vi "gate sts with temp.vi"() -> ()   [LabVIEW 2010]
uses:
  <userlib>/Nanonis Prog Interface V5/Nanonis Prog Interface.lvlib
panel:
  out "Current Gate Voltage (V)":dbl
  out "Ender":bool
  out "Stop Loop":bool
  in  "Stop":bool
  in  "Increment Gate (V)":dbl
  in  "End Gate (V)":dbl
  in  "Start Gate (V)":dbl
  in  "Basename":string
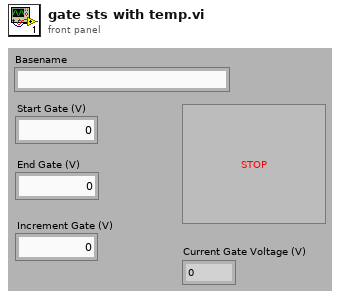
[diagram p1: front panel]
types:
  T1 = cluster{"Save all":enum16{"no change", "on", "off"}, "Number of Sweeps (0=no change)":i32}
  T2 = enum16{"Set Heater Voltage", "Read Heater Voltage", "Read Heater Current", "Read 1K Pot Temperature", "Read IVC Sorb Temperature", "Read Needle Valve Temperature", "Read Still Pressure", "Read Mixing Chamber Temperature", "Read STM RX Temperature", "Read STM CX Temperature", "Unstall Triton Loop", "Triton Stop", "Triton Stall Status"}
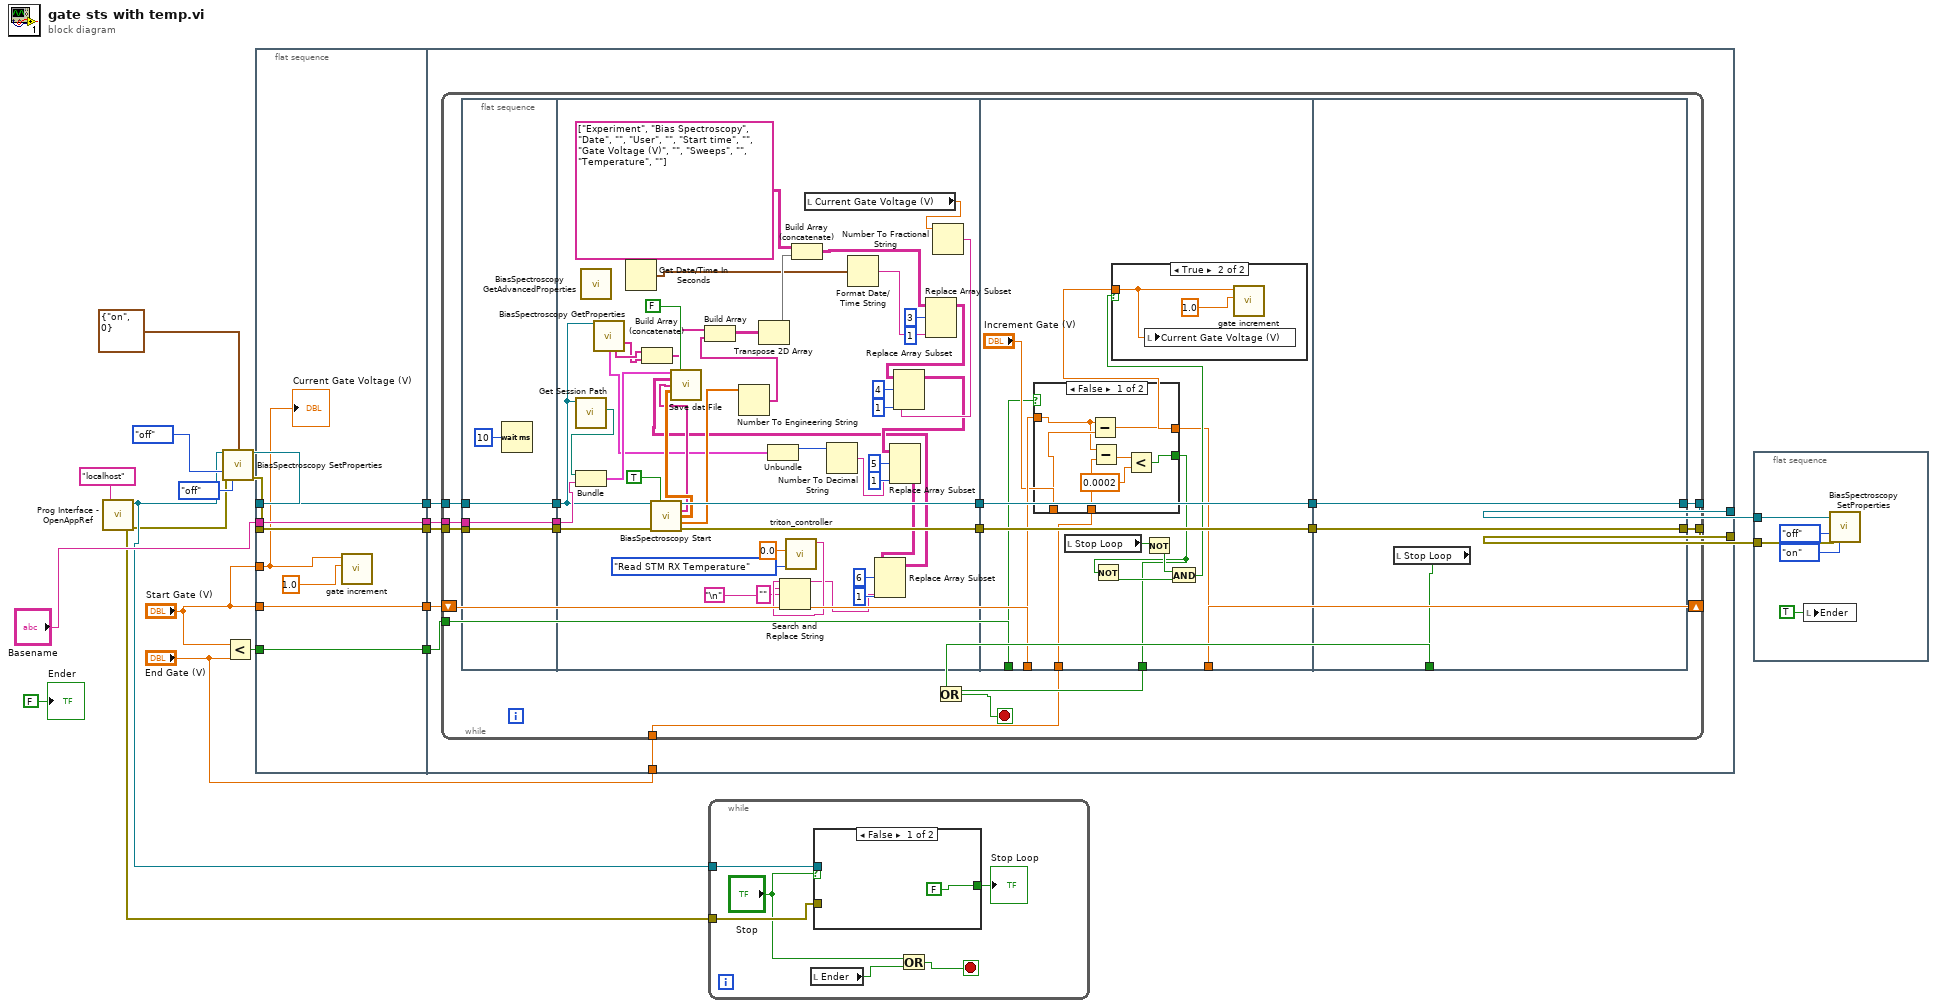
[diagram p0: block diagram]
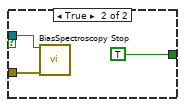
[diagram p2: hidden frame]
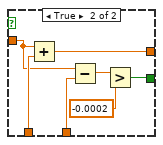
[diagram p3: hidden frame]
diagram:
  n1 = call <userlib>:"Prog Interface - OpenAppRef.vi"("Machine name (local machine IP)"="localhost" ("machine name (localhost)")) -> ("Error out"=w3:errorcluster, "Application reference"=w4:refnum<vi>)  [unwired: 5 in]
  n2 = call <userlib>:"BiasSpectroscopy SetProperties.vi"("Application ref in"=w4, "Autosave (no change)"=enum16{"no change", "on", "off"}."off", "Error in (no error)"=w3, "Save dialog"=enum16{"no change", "on", "off"}."off", "Multiple sweeps config"=T1 {"Save all"=enum."on", "Number of Sweeps (0=no change)"=0}) -> ("Application ref out"=w17:refnum<vi>, "Error out"=w18:errorcluster)  [unwired: 9 in]
  n3 = Less?(x="Start Gate (V)", y="End Gate (V)") -> (x < y?=w12:bool)
  n4 = flat-sequence {
    tunnel: "Start Gate (V)" -> [w23]
    tunnel: w12 -> [w24]
    tunnel: w17 -> [w25]
    tunnel: w18 -> [w26]
    tunnel: "Basename" -> [w27]
    tunnel: [w27] -> w11
    tunnel: [w26] -> w10
    tunnel: [w25] -> w9
    tunnel: [w24] -> w8
    tunnel: [w23] -> w7
    tunnel: "Start Gate (V)" -> [w21]
    tunnel: [w32] -> w15
    tunnel: [w31] -> w14
    tunnel: w11 -> [w35]
    tunnel: w10 -> [w34]
    tunnel: w9 -> [w33]
    tunnel: w8 -> [w30]
    tunnel: w7 -> [w29]
    tunnel: "End Gate (V)" -> [w28]
    frame #0 {
      n5 = call "gate increment.vi"("Increment"=1.0, "Gate Voltage"=w21) -> ()  [unwired: 10 in]
      "Current Gate Voltage (V)" <- w21
    }
    frame #1 {
      n6 = while {
        tunnel: w35 -> [w54]
        tunnel: w34 -> [w53]
        tunnel: w33 -> [w52]
        tunnel: [w51] -> w32
        tunnel: [w50] -> w31
        tunnel: w30 -> [w36]
        shift-right: [w40] -> _
        shift-left: w29 -> [w38]
        tunnel: w28 -> [w37]
        stop <- w41 stop-if-true
        n7 = flat-sequence {
          tunnel: w52 -> [w56]
          tunnel: w53 -> [w57]
          tunnel: w54 -> [w58]
          tunnel: [w58] -> w45
          tunnel: [w57] -> w44
          tunnel: [w56] -> w43
          tunnel: [w101] -> w47
          tunnel: [w102] -> w46
          tunnel: w45 -> [w94]
          tunnel: w44 -> [w103]
          tunnel: w43 -> [w93]
          tunnel: [w115] -> w49
          tunnel: [w114] -> w48
          tunnel: w47 -> [w115]
          tunnel: w46 -> [w114]
          tunnel: [w110] -> w40
          tunnel: [w108] -> w39
          tunnel: w38 -> [w107]
          tunnel: w37 -> [w105]
          tunnel: w36 -> [w104]
          tunnel: [w133] -> w51
          tunnel: [w134] -> w50
          tunnel: w49 -> [w134]
          tunnel: w48 -> [w133]
          tunnel: [w132] -> w42
          frame #0 {
            n8 = Wait (ms)(milliseconds to wait=u32 10) -> ()  [unwired: 1 out]
          }
          frame #1 {
            n9 = call <userlib>:"Get Session Path.vi"("Application ref in"=w93) -> ("Session path"=w99:path)  [unwired: 8 in, 2 out]
            n10 = Bundle("Session path"=w99, "Basename"=w94) -> (w98:cluster{"Session path":path, "Basename":string})  [unwired: 1 in]
            n11 = call <userlib>:"BiasSpectroscopy GetAdvancedProperties.vi"() -> ()  [unwired: 10 in, 6 out]
            n12 = call <userlib>:"BiasSpectroscopy GetProperties.vi"("Application ref in"=w93) -> ("Parameters"=w85:string[], "Multiple sweeps configuration"=w74:cluster{"Number of Sweeps":i32, "Save all":bool}, "Fixed parameters"=w86:string[])  [unwired: 7 in, 5 out]
            n13 = Get Date/Time In Seconds() -> (seconds since 1Jan1904=w84:timestamp)
            n14 = Build Array (concatenate)(w86, w85) -> (w90:string[])
            n15 = call <userlib>:"BiasSpectroscopy Start.vi"("Application ref in"=w93, "Get data (F)"=TRUE, "Error in (no error)"=w103) -> ("Application ref out"=w102:refnum<vi>, "Channels"=w96:string[], "Data"=w97:sgl[][], "Parameters"=w92:sgl[], "Error out"=w101:errorcluster)  [unwired: 8 in]
            n16 = Number To Engineering String(4:w92) -> (0:w91:string[])  [unwired: 3 in]
            n17 = Build Array(w90, w91) -> (w89:string[][])
            n18 = Transpose 2D Array(2D array=w89) -> (transposed array=w87:string[][])
            n19 = Unbundle(w74) -> ("Number of Sweeps"=w73:i32)  [unwired: 1 out]
            n20 = call "triton_controller.vi"("Numerical Argument"=0.0, "Command"=T2."Read STM RX Temperature") -> ("Response"=w62:string)  [unwired: 9 in]
            n21 = Search and Replace String(input string=w62, search string="\n", replace string="" ("replace string (\"\")")) -> (result string=w59:string)  [unwired: 5 in, 3 out]
            n22 = Build Array (concatenate)(string[][] [["Experiment", "Bias Spectroscopy"], ["Date", ""], ["User", ""], ["Start time", ""], ["Gate Voltage (V)", ""], ["Sweeps", ""], ["Temperature", ""]] ("Attributes"), w87) -> (w83:string[][])
            n23 = local read "Current Gate Voltage (V)"() -> (w76:dbl)
            n24 = Number To Decimal String(number=w73) -> (decimal integer string=w69:string)  [unwired: 1 in]
            n25 = Format Date/Time String(seconds (now)=w84) -> (date/time string=w82:string)  [unwired: 2 in]
            n26 = Replace Array Subset(array=w83, new element=w82, index (row)=3, index (col)=1 ("disabled index (col)")) -> (w79:string[][])
            n27 = Number To Fractional String(number=w76) -> (F-format string=w75:string)  [unwired: 3 in]
            n28 = Replace Array Subset(array=w79, new element=w75, index (row)=4, index (col)=1 ("disabled index (col)")) -> (w72:string[][])
            n29 = Replace Array Subset(array=w72, new element=w69, index (row)=5, index (col)=1 ("disabled index (col)")) -> (w64:string[][])
            n30 = Replace Array Subset(array=w64, new element=w59, index (row)=6, index (col)=1) -> (w63:string[][])
            n31 = call <userlib>:"Save dat File.vi"("Filename control"=w98, "Show save dialog (T)"=FALSE, "Attributes"=w63, "Channels names"=w96, "Data"=w97) -> ()  [unwired: 7 in, 4 out]
          }
          frame #2 {
            n32 = case shown="False" w104 {
              tunnel: w107 -> [w120 w126]
              tunnel: "Increment Gate (V)" -> [w121 w129]
              tunnel: [w122 w128] -> w110
              tunnel: w105 -> [w119 w127]
              tunnel: [w117 w125] -> w108
              frame False {
                n33 = Subtract(x=w120, y=w121) -> (x-y=w122:dbl)
                n34 = Subtract(x=w120, y=w119) -> (x-y=w118:dbl)
                n35 = Less?(x=w118, y=0.0002) -> (x < y?=w117:bool)
              }
              frame True {
                n36 = Add(x=w126, y=w129) -> (x+y=w128:dbl)
                n37 = Subtract(x=w126, y=w127) -> (x-y=w124:dbl)
                n38 = Greater?(x=w124, y=-0.0002) -> (0:w125:bool)
              }
            }
            n39 = local read "Stop Loop"() -> (w113:bool)
            n40 = Not(x=w108) -> (.not. x?=w109:bool)
            n41 = Not(x=w113) -> (.not. x?=w111:bool)
            n42 = And(x=w111, y=w109) -> (x .and. y?=w112:bool)
            n43 = case shown="True" w112 {
              tunnel: w110 -> [_ w131]
              frame False {
              }
              frame True {
                n44 = local write "Current Gate Voltage (V)"(w131) -> ()
                n45 = call "gate increment.vi"("Increment"=1.0, "Gate Voltage"=w131) -> ()  [unwired: 10 in]
              }
            }
          }
          frame #3 {
            n46 = local read "Stop Loop"() -> (w132:bool)
          }
        }
        n47 = Or(x=w39, y=w42) -> (x .or. y?=w41:bool)
      }
    }
  }
  n48 = while {
    tunnel: w4 -> [w140]
    tunnel: w3 -> [w139]
    stop <- w136 stop-if-true
    n49 = local read "Ender"() -> (w135:bool)
    n50 = case shown="False" "Stop" {
      tunnel: w140 -> [_ w144]
      tunnel: w139 -> [_ w143]
      tunnel: [FALSE TRUE] -> w138
      frame False {
      }
      frame True {
        n51 = call <userlib>:"BiasSpectroscopy Stop.vi"("Application ref in"=w144, "Error in (no error)"=w143) -> ()  [unwired: 12 in, 2 out]
      }
    }
    "Stop Loop" <- w138
    n52 = Or(x="Stop", y=w135) -> (x .or. y?=w136:bool)
  }
  n53 = flat-sequence {
    tunnel: w15 -> [w149]
    tunnel: w14 -> [w148]
    frame #0 {
      n54 = local write "Ender"(TRUE ("Ender")) -> ()
      n55 = call <userlib>:"BiasSpectroscopy SetProperties.vi"("Application ref in"=w149, "Autosave (no change)"=enum16{"no change", "on", "off"}."off", "Error in (no error)"=w148, "Save dialog"=enum16{"no change", "on", "off"}."on") -> ()  [unwired: 10 in, 2 out]
    }
  }
  "Ender" <- FALSE ("Ender")
